vi "handle minute ave.vi"(11 "Array":dbl[](array[numeric])) -> (0 "Correct":bool, 3 "Array 2":i32[](array[numeric]))   [LabVIEW 2019]
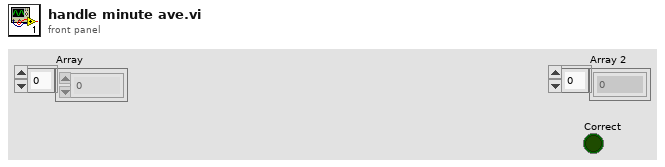
[diagram p1: front panel]
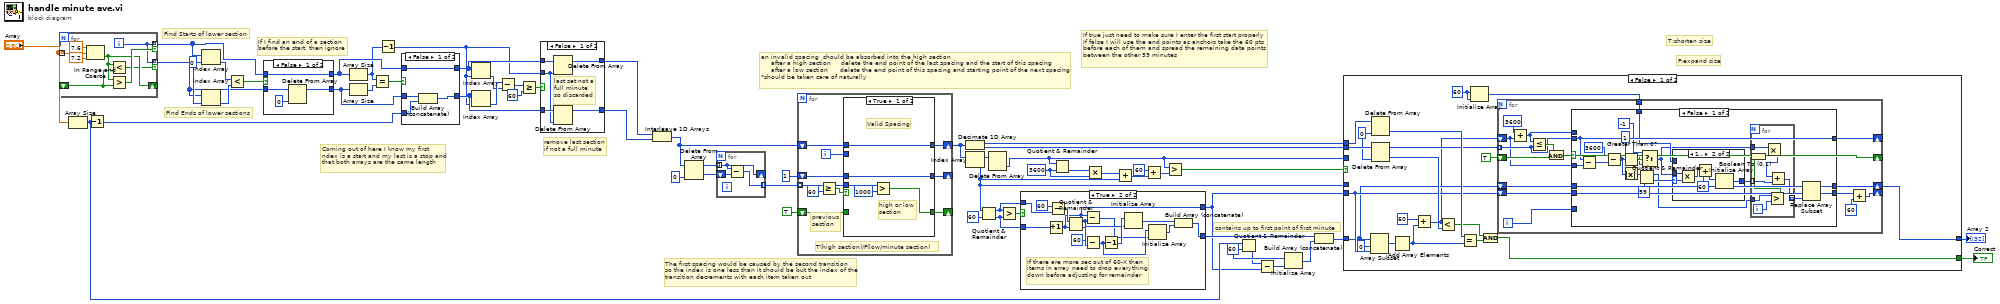
[diagram p0: block diagram]
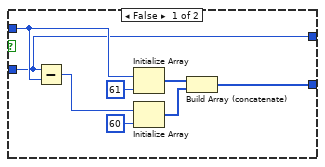
[diagram p2: hidden frame]
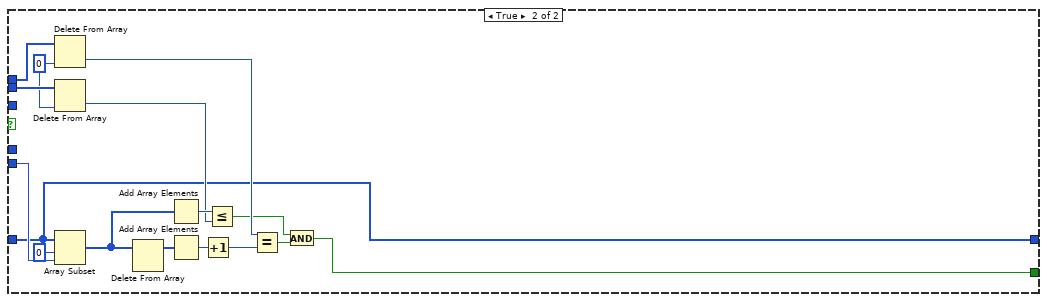
[diagram p5: hidden frame]
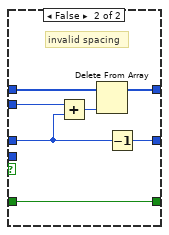
[diagram p6: hidden frame]
diagram:
  w9 = 3600 ("y")
  w19 = 60 ("y")
  w56 = 0 ("index")
  # "T:shorten size"
  # "F:expand size"
  # "contains up to first point of first minute"
  # "If true just need to make sure I enter the first start properly\nIf false I will use the end points as anchors take the 60 pts\nbefore each of them and spread the remaining data points\nbetween the other 59 minutes"
  # "The first spacing would be caused by the second transition\nso the index is one less than it should be but the index of the\ntransition decrements with each item taken out"
  # "an invalid spacing  should be absorbed into the high section\n     after a high section     delete the end point of the last spacing and the start of this spacing\n     after a low section      delete the end point of this spacing and starting point of the next spacing\n*should be taken care of naturally"
  # "remove last section\nif not a full minute"
  # "If I find an end of a section\nbefore the start, then ignore"
  # "Coming out of here I know my first \nndex is a start and my last is a stop and\nthat both arrays are the same length"
  # "Find Ends of lower sections"
  # "Find Starts of lower section"
  n1 = for {
    tunnel: "Array" -> [w64] mode=indexing
    tunnel: [w58] -> w52 mode=indexing if=w61
    shift-right: [w60] -> _
    shift-left: _ -> [w59]
    tunnel: [w58] -> w51 mode=indexing if=w57
    i -> [w58]
    n2 = In Range and Coerce(upper limit=7.6, x=w64, lower limit=7.2) -> (In Range?=w60:bool)  [unwired: 1 out]
    n3 = Less?(x=w60, y=w59) -> (x < y?=w57:bool)
    n4 = Greater?(x=w60, y=w59) -> (0:w61:bool)
  }
  n5 = Array Size(array="Array") -> (size(s)=w24:i32)
  n6 = Decrement(x=w24) -> (x-1=w46:i32)
  n7 = Index Array(array=w52, index=w56) -> (element=w55:i32)
  n8 = Index Array(array=w51, index=w56) -> (element=w54:i32)
  n9 = Less?(x=w55, y=w54) -> (x < y?=w53:bool)
  n10 = case shown="False" w53 {
    tunnel: w52 -> [w68 w70]
    tunnel: w51 -> [w67 w69]
    tunnel: [w68 w70] -> w48
    tunnel: [w66 w69] -> w47
    frame False {
      n11 = Delete From Array(array=w67, index=0) -> (array with subset deleted=w66:i32[])  [unwired: 1 in, 1 out]
    }
    frame True {
    }
  }
  n12 = Array Size(array=w48) -> (size(s)=w44:i32)
  n13 = Array Size(array=w47) -> (size(s)=w45:i32)
  n14 = Equal?(x=w44, y=w45) -> (x = y?=w49:bool)
  n15 = Decrement(x=w44) -> (x-1=w36:i32)
  n16 = case shown="False" w49 {
    tunnel: w48 -> [w72 w76]
    tunnel: w47 -> [w74 w75]
    tunnel: w46 -> [w73 _]
    tunnel: [w72 w76] -> w38
    tunnel: [w71 w75] -> w37
    frame False {
      n17 = Build Array (concatenate)(w74, w73) -> (w71:i32[])
    }
    frame True {
    }
  }
  n18 = Index Array(array=w38, index=w36) -> (element=w42:i32)
  n19 = Index Array(array=w37, index=w36) -> (element=w43:i32)
  n20 = Subtract(x=w43, y=w42) -> (x-y=w41:i32)
  n21 = Greater Or Equal?(x=w41, y=60) -> (x >= y?=w39:bool)
  n22 = case shown="False" w39 {
    tunnel: w38 -> [w80 w83]
    tunnel: w37 -> [w81 w82]
    tunnel: [w79 w83] -> w35
    tunnel: [w78 w82] -> w34
    tunnel: w36 -> [w77 _]
    frame False {
      # "last set not a\nfull minute\nso discarded"
      n23 = Delete From Array(array=w80, index=w77) -> (array with subset deleted=w79:i32[])  [unwired: 1 in, 1 out]
      n24 = Delete From Array(array=w81, index=w77) -> (array with subset deleted=w78:i32[])  [unwired: 1 in, 1 out]
    }
    frame True {
      # "last set has a\nminute of data"
    }
  }
  n25 = Interleave 1D Arrays(w35, w34) -> (w28:i32[])
  n26 = Delete From Array(array=w28, index=0) -> (deleted portion=w32:i32, array with subset deleted=w31:i32[])  [unwired: 1 in]
  n27 = for {
    tunnel: w31 -> [w85] mode=indexing
    shift-right: [w85] -> _
    shift-left: w32 -> [w86]
    tunnel: [w84] -> w30 mode=indexing
    n28 = Subtract(x=w85, y=w86) -> (x-y=w84:i32)
  }
  n29 = for {
    tunnel: w30 -> [w93] mode=indexing
    shift-right: [w94] -> _
    shift-left: TRUE -> [w95]
    shift-right: [w90] -> w26
    shift-left: w28 -> [w91]
    shift-right: [w87] -> _
    shift-left: 1 -> [w88]
    i -> [w89]
    # "previous\nsection"
    # "T(high section)/F(low/minute section)"
    n30 = Greater Or Equal?(x=w93, y=60) -> (x >= y?=w92:bool)
    n31 = case shown="True" w92 {
      tunnel: w95 -> [_ w108]
      tunnel: [w99 w108] -> w94
      tunnel: w93 -> [w100 _]
      tunnel: w91 -> [w98 w107]
      tunnel: [w98 w106] -> w90
      tunnel: w89 -> [_ w103]
      tunnel: w88 -> [w97 w105]
      tunnel: [w97 w104] -> w87
      frame True {
        # "high or low\nsection"
        # "Valid Spacing"
        n32 = Greater?(x=w100, y=1000) -> (0:w99:bool)
      }
      frame False {
        # "invalid spacing"
        n33 = Add(x=w103, y=w105) -> (x+y=w102:i32)
        n34 = Delete From Array(array=w107, index=w102) -> (array with subset deleted=w106:i32[])  [unwired: 1 in, 1 out]
        n35 = Decrement(x=w105) -> (x-1=w104:i32)
      }
    }
  }
  n36 = Decimate 1D Array(w26) -> (w25:i32[], w13:i32[])
  n37 = Index Array(array=w26) -> (element=w6:i32)  [unwired: 1 in]
  n38 = Quotient & Remainder(x=w6, y=60) -> (x-y*floor(x/y)=w21:i32, floor(x/y)=w20:i32)
  n39 = Delete From Array(array=w26) -> (deleted portion=w4:i32)  [unwired: 2 in, 1 out]
  n40 = Greater?(x=w21, y=w20) -> (0:w22:bool)
  n41 = case shown="True" w22 {
    tunnel: w21 -> [w116 w129]
    tunnel: w20 -> [w109 w130]
    tunnel: [w110 w118] -> w16
    tunnel: [w109 w117] -> w15
    frame False {
      n42 = Subtract(x=w109, y=w116) -> (x-y=w115:i32)
      n43 = Initialize Array(w116, 61 ("dimension size")) -> (w112:i32[])
      n44 = Initialize Array(w115, 60 ("dimension size")) -> (w111:i32[])
      n45 = Build Array (concatenate)(w112, w111) -> (w110:i32[])
    }
    frame True {
      # "If there are more sec out of 60-X then\nitems in array need to drop everything\ndown before adjusting for remainder"
      n46 = Increment(x=w130) -> (x+1=w117:i32)
      n47 = Subtract(x=60, y=w129) -> (x-y=w127:i32)
      n48 = Quotient & Remainder(x=w127, y=w117) -> (x-y*floor(x/y)=w122:i32, floor(x/y)=w126:i32)
      n49 = Subtract(x=w117, y=w122) -> (x-y=w121:i32)
      n50 = Subtract(x=60, y=w126) -> (x-y=w124:i32)
      n51 = Decrement(x=w124) -> (x-1=w123:i32)
      n52 = Initialize Array(w123, w122) -> (w120:i32[])
      n53 = Initialize Array(w124, w121) -> (w119:i32[])
      n54 = Build Array (concatenate)(w120, w119) -> (w118:i32[])
    }
  }
  n55 = Quotient & Remainder(x=w4, y=w9) -> (floor(x/y)=w10:i32)  [unwired: 1 out]
  n56 = Multiply(x=w10, y=w9) -> (x*y=w8:i32)
  n57 = Add(x=w8, y=w6) -> (x+y=w7:i32)
  n58 = Add(x=60, y=w7) -> (x+y=w3:i32)
  n59 = Greater?(x=w4, y=w3) -> (0:w2:bool)
  n60 = Quotient & Remainder(x=w24, y=w19) -> (floor(x/y)=w12:i32)  [unwired: 1 out]
  n61 = Subtract(x=w12, y=w15) -> (x-y=w18:i32)
  n62 = Initialize Array(w19, w18) -> (w17:i32[])
  n63 = Build Array (concatenate)(w16, w17) -> (w14:i32[])
  n64 = case shown="False" w2 {
    tunnel: w6 -> [_ _]
    tunnel: w4 -> [_ _]
    tunnel: w25 -> [w148 w213]
    tunnel: w15 -> [w140 w219]
    tunnel: w14 -> [w139 w205]
    tunnel: [w135 w205] -> w11
    tunnel: w13 -> [w147 w212]
    tunnel: [w134 w204] -> w1
    frame False {
      w137 = 60 ("y")
      w146 = 0 ("index")
      n65 = Array Subset(array=w139, index=0, length=w140) -> (w149:i32[])
      n66 = Delete From Array(array=w148, index=w146) -> (deleted portion=w145:i32)  [unwired: 1 in, 1 out]
      n67 = Delete From Array(array=w147, index=w146) -> (deleted portion=w144:i32, array with subset deleted=w141:i32[])  [unwired: 1 in]
      n68 = Add Array Elements(numeric array=w149) -> (sum=w133:i32)
      n69 = Add(x=60, y=w133) -> (x+y=w131:i32)
      n70 = Less?(x=w131, y=w144) -> (x < y?=w143:bool)
      n71 = Equal?(x=w145, y=w133) -> (x = y?=w142:bool)
      n72 = Initialize Array(w137, w137) -> (w136:i32[])
      n73 = And(x=w143, y=w142) -> (x .and. y?=w134:bool)
      n74 = for {
        tunnel: w141 -> [w161] mode=indexing
        shift-right: [w154] -> _
        shift-left: w140 -> [w158]
        shift-right: [w159] -> w135
        shift-left: w139 -> [w160]
        shift-right: [w162] -> _
        shift-left: w131 -> [w157]
        shift-right: [w153] -> _
        shift-left: TRUE -> [w164]
        tunnel: w136 -> [w152]
        i -> [w151]
        n75 = Add(x=3600, y=w157) -> (x+y=w163:i32)
        n76 = Less Or Equal?(x=w163, y=w161) -> (x <= y?=w165:bool)
        n77 = And(x=w165, y=w164) -> (x .and. y?=w153:bool)
        n78 = case shown="False" w153 {
          tunnel: w163 -> [_ w203]
          tunnel: [w182 w203] -> w162
          tunnel: w161 -> [w182 _]
          tunnel: w160 -> [w185 w202]
          tunnel: [w184 w202] -> w159
          tunnel: w158 -> [w183 w201]
          tunnel: w157 -> [w181 _]
          tunnel: [w183 w201] -> w155
          tunnel: w152 -> [w178 _]
          tunnel: w151 -> [_ _]
          frame False {
            n79 = Subtract(x=w182, y=w181) -> (x-y=w179:i32)
            n80 = Subtract(x=3600, y=w179) -> (x-y=w176:i32)
            n81 = Greater Than 0?(x=w176) -> (x > 0?=w173:bool)
            n82 = Absolute Value(x=w176) -> (abs(x)=w177:i32)
            n83 = Quotient & Remainder(x=w177, y=59) -> (x-y*floor(x/y)=w168:i32, floor(x/y)=w174:i32)
            n84 = Select(t=-1 ("y"), s=w173, f=1 ("y")) -> (s? t:f=w169:i32)
            n85 = case shown="1.." w174 {
              selector: w174 -> [_ w197]
              tunnel: w178 -> [w194 _]
              tunnel: [w194 w198] -> w170
              tunnel: w169 -> [_ w195]
              frame 0, Default {
              }
              frame 1.. {
                w200 = 60 ("y")
                n86 = Multiply(x=w195, y=w197) -> (x*y=w196:i32)
                n87 = Add(x=w196, y=w200) -> (x+y=w199:i32)
                n88 = Initialize Array(w199, w200) -> (w198:i32[])
              }
            }
            n89 = for {
              tunnel: w170 -> [w189] mode=indexing
              tunnel: w169 -> [w191]
              tunnel: w168 -> [w193]
              tunnel: [w187] -> w167 mode=indexing
              i -> [w192]
              n90 = Greater?(x=w193, y=w192) -> (0:w186:bool)
              n91 = Boolean To (0,1)(Boolean=w186) -> (0, 1=w190:i16)
              n92 = Multiply(x=w191, y=w190) -> (x*y=w188:i32)
              n93 = Add(x=w188, y=w189) -> (x+y=w187:i32)
            }
            n94 = Replace Array Subset(array=w185, new element=w167, index=w183) -> (w184:i32[])
          }
          frame True {
          }
        }
        n95 = Add(x=w155, y=60) -> (x+y=w154:i32)
      }
    }
    frame True {
      w211 = 0 ("index")
      n96 = Delete From Array(array=w213, index=w211) -> (deleted portion=w210:i32)  [unwired: 1 in, 1 out]
      n97 = Delete From Array(array=w212, index=w211) -> (deleted portion=w208:i32)  [unwired: 1 in, 1 out]
      n98 = Array Subset(array=w205, index=0, length=w219) -> (w216:i32[])
      n99 = Delete From Array(array=w216) -> (array with subset deleted=w217:i32[])  [unwired: 2 in, 1 out]
      n100 = Add Array Elements(numeric array=w216) -> (sum=w209:i32)
      n101 = Add Array Elements(numeric array=w217) -> (sum=w215:i32)
      n102 = Increment(x=w215) -> (x+1=w214:i32)
      n103 = Less Or Equal?(x=w209, y=w208) -> (x <= y?=w207:bool)
      n104 = Equal?(x=w210, y=w214) -> (x = y?=w206:bool)
      n105 = And(x=w207, y=w206) -> (x .and. y?=w204:bool)
    }
  }
  "Correct" <- w1
  "Array 2" <- w11
